vi "topicRequest.vi"(1 "XML":string) -> (0 "Subscriber":T1)   [LabVIEW 2013]
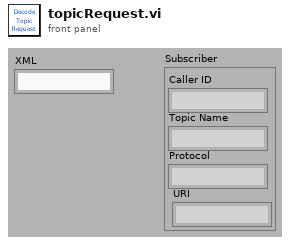
[diagram p1: front panel]
types:
  T1 = cluster{"Caller ID":string, "Topic Name":string, "Protocol":string, "URI":string}
  T2 = cluster{"Caller ID":string, "Topic Name":string, "Protocol":string, "Caller ID 2":string}
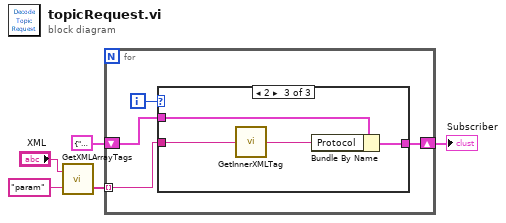
[diagram p0: block diagram]
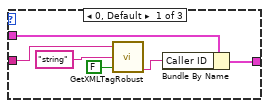
[diagram p2: hidden frame]
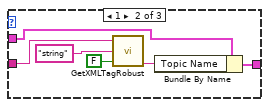
[diagram p3: hidden frame]
diagram:
  n1 = call "GetXMLArrayTags.vi"("ArrayTag"="param", "String"="XML") -> ("Array"=w3:string[])  [unwired: 1 out]
  n2 = for {
    tunnel: w3 -> [w7] mode=indexing
    shift-right: [w6] -> w5
    shift-left: T2 {"Caller ID"="", "Topic Name"="", "Protocol"="", "Caller ID 2"=""} ("Subscriber") -> [w8]
    i -> [w9]
    n3 = case shown="2" w9 {
      tunnel: w8 -> [w13 w21 w23]
      tunnel: w7 -> [w15 w19 w25]
      tunnel: [w11 w20 w22] -> w6
      frame 0, Default {
        n4 = call "GetXMLTagRobust.vi"("Tag only? (T)"=FALSE ("Tag only?"), "Tag"="string", "String"=w15) -> ("value"=w12:string)  [unwired: 3 out]
        n5 = Bundle By Name(cluster=w13, "Caller ID"=w12) -> (w11:T2)
      }
      frame 1 {
        n6 = call "GetXMLTagRobust.vi"("Tag only? (T)"=FALSE ("Tag only?"), "Tag"="string", "String"=w19) -> ("value"=w16:string)  [unwired: 3 out]
        n7 = Bundle By Name(cluster=w21, "Topic Name"=w16) -> (w20:T2)
      }
      frame 2 {
        n8 = call "GetInnerXMLTag.vi"("String"=w25) -> ("Value"=w24:string)
        n9 = Bundle By Name(cluster=w23, "Protocol"=w24) -> (w22:T2)
      }
    }
  }
  "Subscriber" <- w5
